vi "SetValue.vi"(7 "error in (no error)":errorcluster, 10 "Value":i32) -> (3 "TestClass out":refnum<class "TestClass.lvclass">, 5 "error out":errorcluster)   [LabVIEW 2013, in "TestClass.lvclass"]
doc: "Provides a Set method for the TestClass"
uses:
  TestClass.lvclass
  TestClass.lvclass/TestClass.ctl
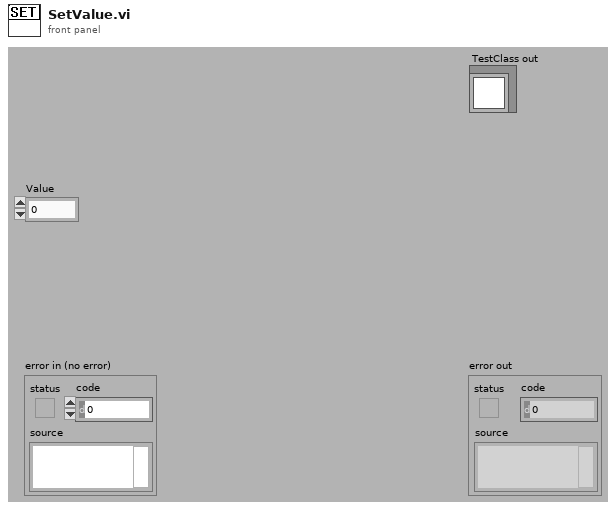
[diagram p1: front panel]
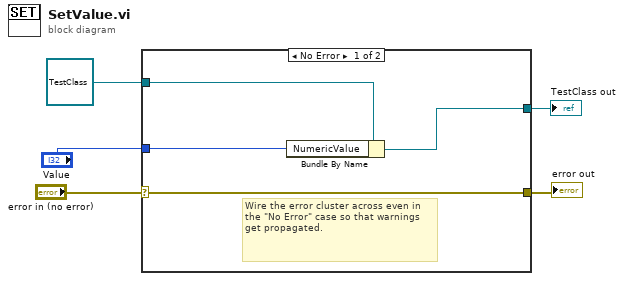
[diagram p0: block diagram]
diagram:
  n1 = case shown="No Error" "error in (no error)" {
    selector: "error in (no error)" -> [w9 w11]
    tunnel: [w9 w11] -> w4
    tunnel: [w8 w10] -> w2
    tunnel: refnum<class "TestClass.lvclass"> refnum ("TestClass in") -> [w7 w10]
    tunnel: "Value" -> [w6 _]
    frame No Error {
      # "Wire the error cluster across even in the \"No Error\" case so that warnings get propagated."
      n2 = Bundle By Name(cluster=w7, "NumericValue"=w6) -> (w8:refnum<class "TestClass.lvclass">)
    }
    frame Error {
    }
  }
  "error out" <- w4
  "TestClass out" <- w2
